vi "Main.vi"(11 "Module Admin":refnum<class "Delacor_lib_QMH_Module Admin.lvclass">) -> ()   [LabVIEW 2021, in "TDMS.lvlib"]
doc: "This template is based off of the Queued Message Handler design pattern and the Queued Message Handler project template that ships with LabVIEW.\n\nThe main difference is that the queue is private to this module and communication between modules is performed via Broadcast and Request events.\n\nRequest events are wrapped in public API methods and are handled in the Event Handling Loop (EHL) of this VI. Any module can register for Broadcast events sent by this module. The EHL generates messages based on user interface actions.\n\nThe Message Handling Loop (MHL) processes messages generated by the EHL, or by other messages. The messages are string values, so new messages can be added easily to the Message Cases case structure in the MHL. Each message cluster can also provide an optional value for Message Data, which is a variant that can be converted to whatever message-specific data is required.\n_____\nBased on DQMH Project Template 7.0.1.1316."
uses:
  TDMS.lvlib
  <vilib>/Delacor/Delacor QMH/Libraries/Module Admin_class/Delacor_lib_QMH_Module Admin.lvclass
  Module Data--cluster.ctl
  Stop Argument--cluster.ctl
  <vilib>/Delacor/Delacor QMH/Libraries/Message Queue_class/Delacor_lib_QMH_Message Queue.lvclass/Delacor_lib_QMH_Message Queue.ctl
  <vilib>/Delacor/Delacor QMH/Libraries/Module Admin_class/Delacor_lib_QMH_Module Admin.lvclass/Delacor_lib_QMH_Module Admin.ctl
  Write Data Argument--cluster.ctl
  RT Main/Data Cluster.ctl
  <vilib>/Delacor/Delacor QMH/Libraries/Message Queue_class/Delacor_lib_QMH_Enqueue Message (Single).vi
  <vilib>/Delacor/Delacor QMH/Libraries/Module Admin_class/Delacor_lib_QMH_Get External Launch.vi
  <vilib>/Delacor/Delacor QMH/Libraries/Message Queue_class/Delacor_lib_QMH_Message Queue.lvclass
  RT Main/RT Main.lvlib
  <vilib>/WebDAVClient/NI_WebDAV.lvlib
  <vilib>/WebDAVClient/Advanced/Get File.vi
panel:
  out "error out":errorcluster
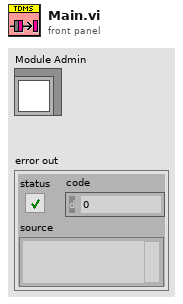
[diagram p1: front panel]
types:
  T1 = typedef "TDMS.lvlib/Request Events--cluster.ctl" = cluster{"Stop Module":refnum<user-event>, "Show Panel":refnum<user-event>, "Hide Panel":refnum<user-event>, "Get Module Execution Status":refnum<user-event>, "Show Diagram":refnum<user-event>, "Create TDMS File":refnum<user-event>, "Close TDMS File":refnum<user-event>, "Write Data":refnum<user-event>, "Private.Write Data to File":refnum<user-event>}
  T2 = typedef "TDMS.lvlib/Module Data--cluster.ctl" = cluster{"Status":string, "Path":path, "tdms file Ref":refnum<k34>}
  T3 = enum32{"invalid lock state", "Not Locked", "Locked (No Password)", "Password-protected"}
  T4 = typedef "TDMS.lvlib/Stop Argument--cluster.ctl" = cluster{"Origin":string, "Exit via Stop Module Req?":bool, "Wait for Module to stop?":bool}
  T5 = typedef "TDMS.lvlib/Write Data Argument--cluster.ctl" = cluster{"Data":T6[]}
  T6 = typedef "RT Main.lvlib/Data Cluster.ctl" = cluster{"Analog Input":dbl[], "Digital Inputs":bool[], "U32":u32[]}
  T7 = enum16{"open", "open or create", "create or replace", "create", "open (read-only)"}
  T8 = typedef "NI_WebDAV.lvlib/SessionHandle.ctl" = refnum<k1>
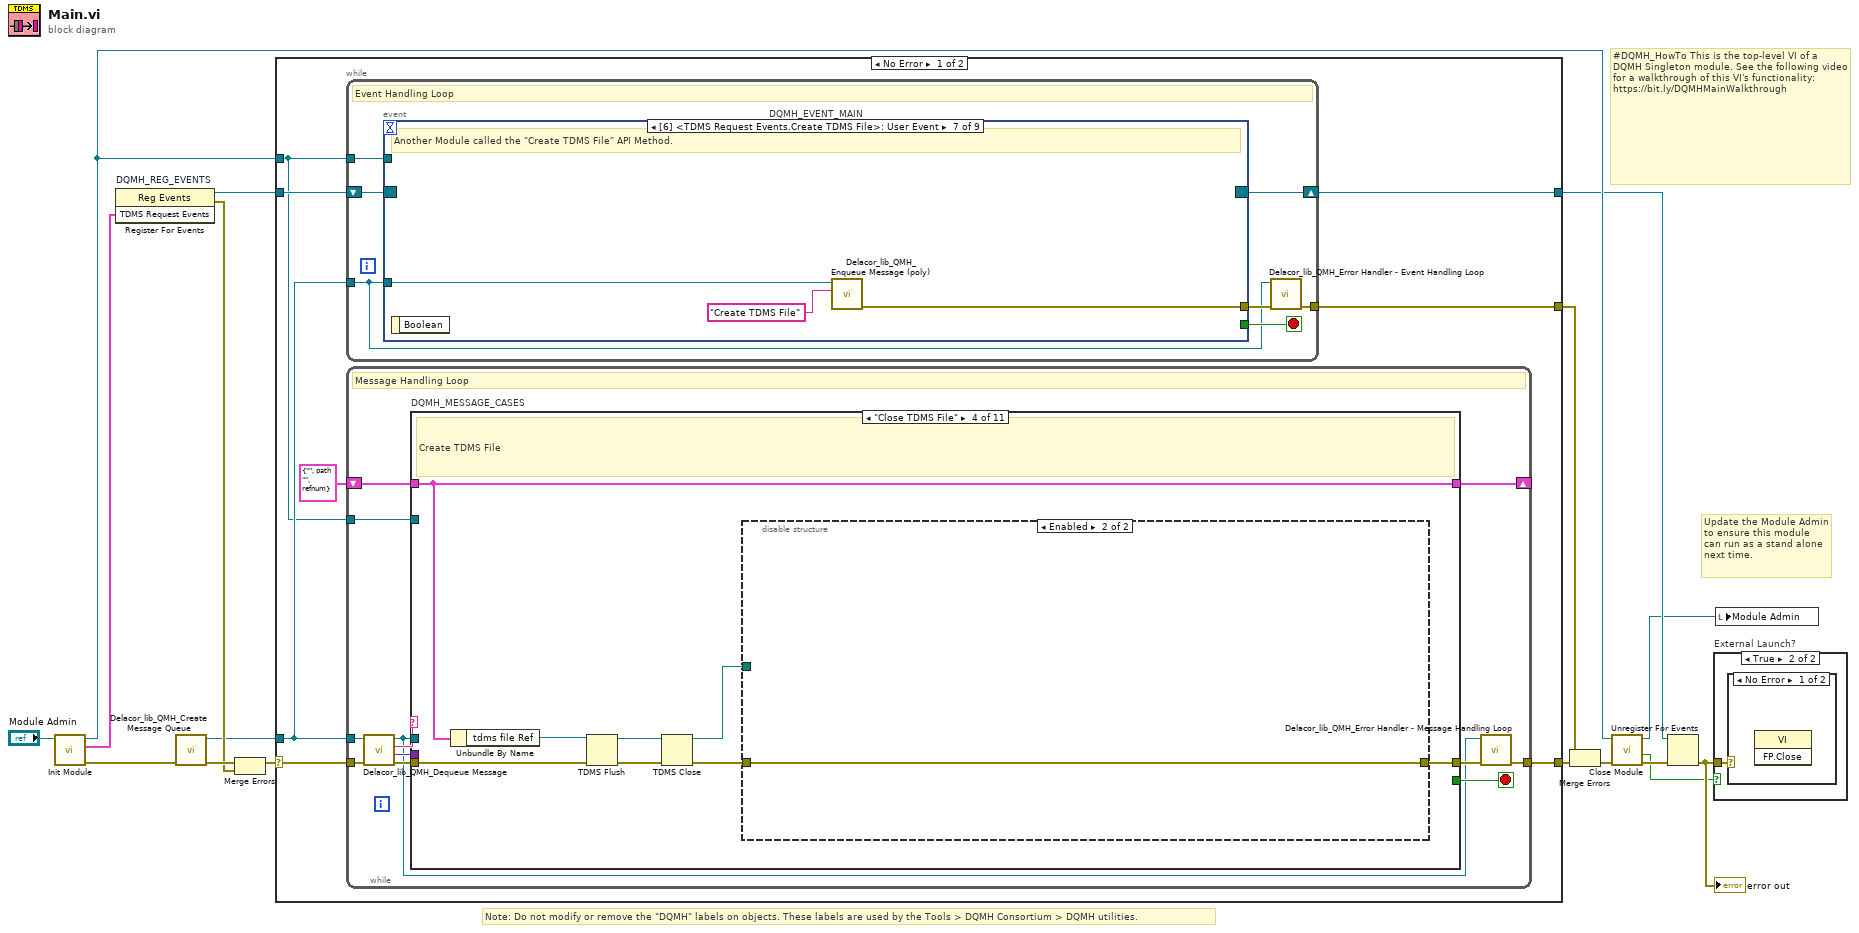
[diagram p0: block diagram]
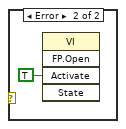
[diagram p3: hidden frame]
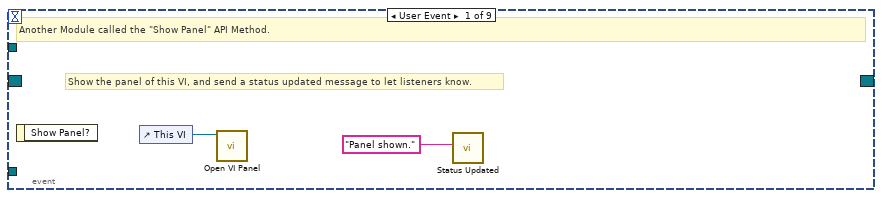
[diagram p4: hidden frame]
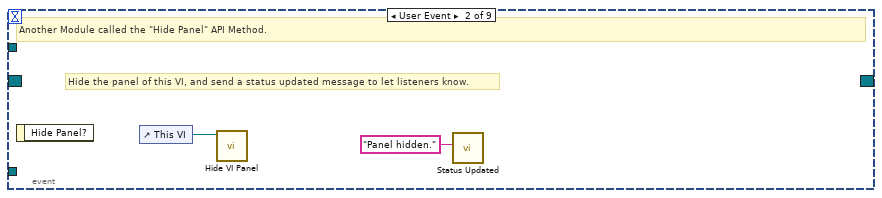
[diagram p5: hidden frame]
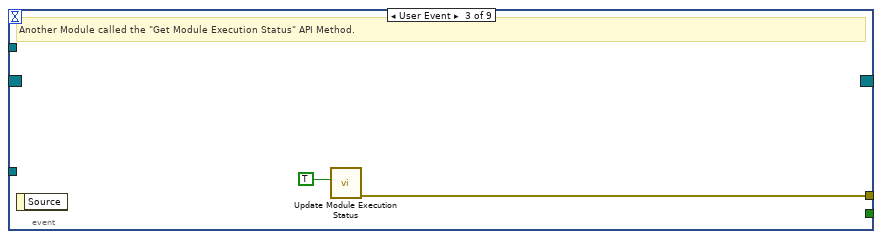
[diagram p6: hidden frame]
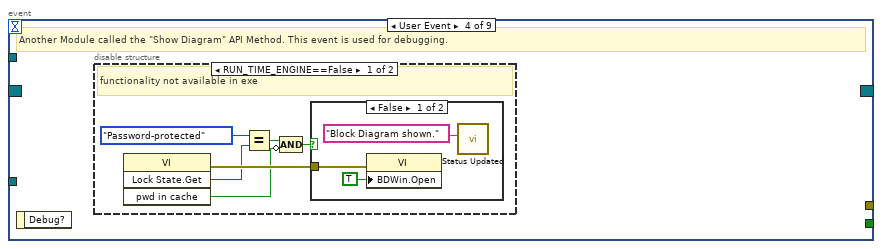
[diagram p7: hidden frame]
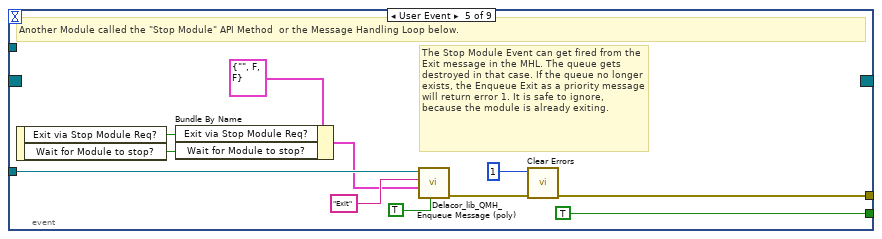
[diagram p10: hidden frame]
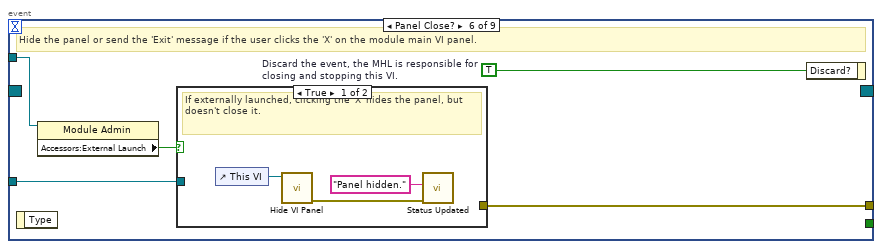
[diagram p11: hidden frame]
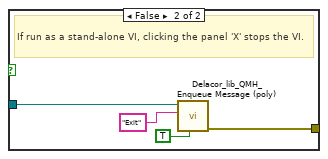
[diagram p12: hidden frame]
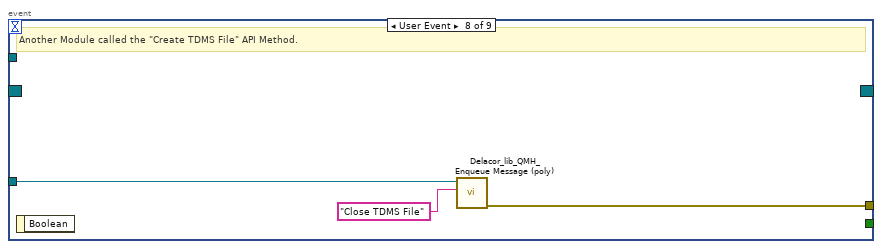
[diagram p13: hidden frame]
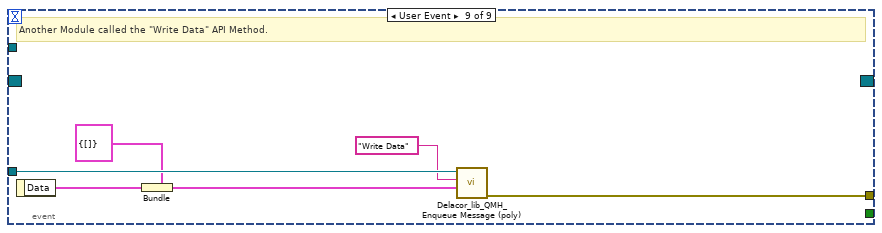
[diagram p14: hidden frame]
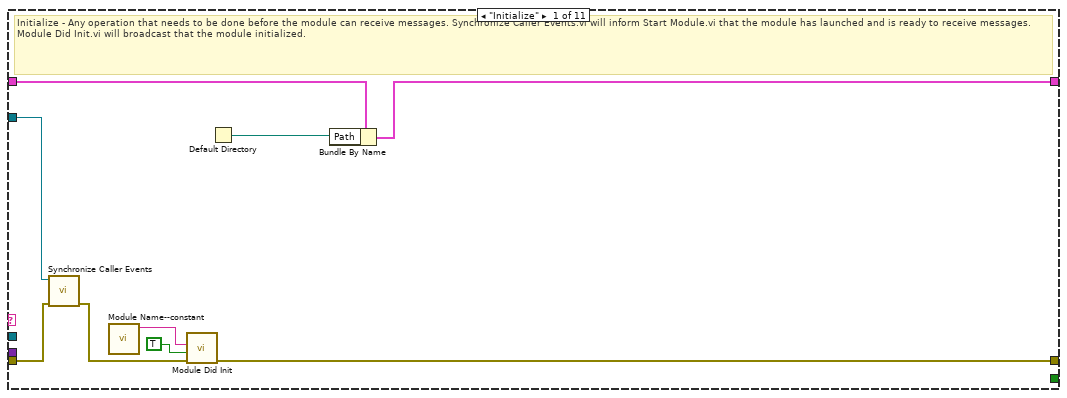
[diagram p15: hidden frame]
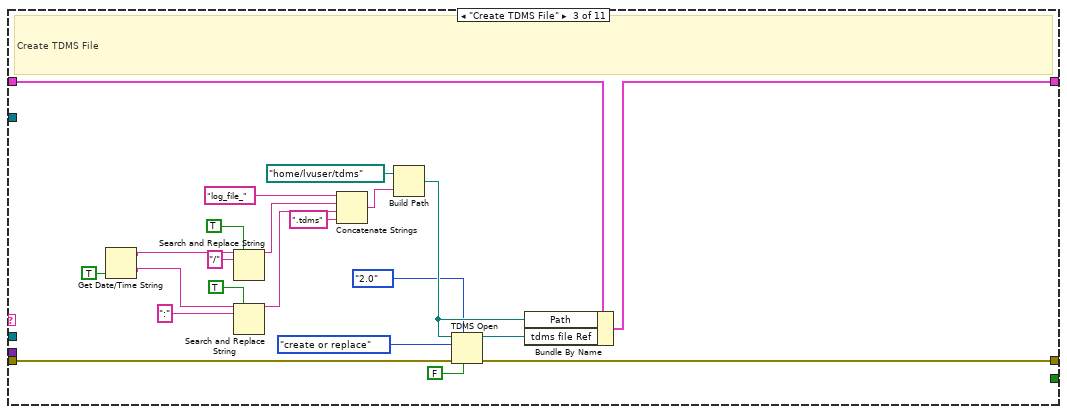
[diagram p17: hidden frame]
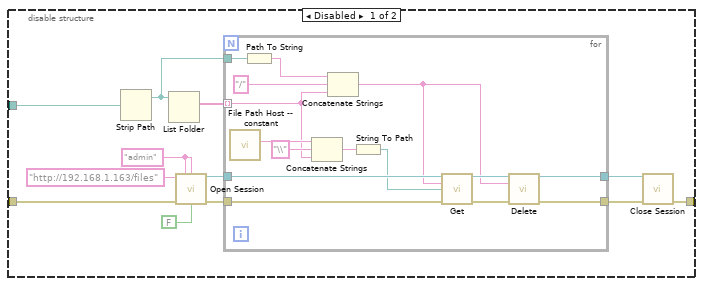
[diagram p18: hidden frame]
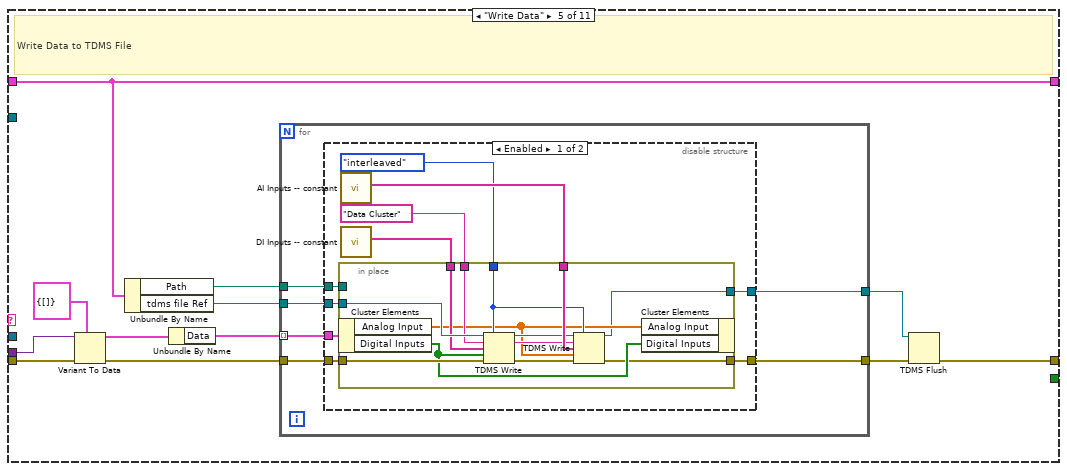
[diagram p19: hidden frame]
diagram:
  # "#DQMH_HowTo This is the top-level VI of a DQMH Singleton module. See the following video for a walkthrough of this VI's functionality: https://bit.ly/DQMHMainWalkthrough"
  # "Note: Do not modify or remove the \"DQMH\" labels on objects. These labels are used by the Tools > DQMH Consortium > DQMH utilities."
  # "Update the Module Admin to ensure this module can run as a stand alone next time."
  n1 = call "Init Module.vi"("Singleton Module Admin in"="Module Admin") -> ("error out"=w16:errorcluster, "TDMS Request Events"=w1:T1, "Singleton Module Admin out"=w8:refnum<class "Delacor_lib_QMH_Module Admin.lvclass">)  [unwired: 8 in]
  n2 = register-events "DQMH_REG_EVENTS"(w1) -> (reference out=w6:refnum<event-registration>, error out=w9:errorcluster)  [unwired: 2 in]
  n3 = call <vilib>:"Delacor_lib_QMH_Create Message Queue.vi"("error in"=w16) -> ("error out"=w11:errorcluster, "Message Queue"=w5:refnum<class "Delacor_lib_QMH_Message Queue.lvclass">)  [unwired: 9 in]
  n4 = Merge Errors(w11, w9) -> (w10:errorcluster)
  n5 = case shown="No Error" w10 {
    selector: w10 -> [w23 w269]
    tunnel: [w25 w268] -> w17
    tunnel: [w22 w267] -> w7
    tunnel: w6 -> [w20 w267]
    tunnel: w5 -> [w19 w262]
    tunnel: [w24 _] -> w14
    tunnel: w8 -> [w18 w263]
    frame No Error {
      n6 = while {
        tunnel: w19 -> [w26]
        shift-right: [w29] -> w22
        shift-left: w20 -> [w30]
        tunnel: [w31] -> w24
        tunnel: w18 -> [w27]
        stop <- w28 stop-if-true
        # "Event Handling Loop"
        n7 = event "DQMH_EVENT_MAIN" shown="[6] <TDMS Request Events.Create TDMS File>: User Event" {
          selector: w30 -> [_ _ _ _ _ _ _ _ _]
          dyn-events: [_ _ _ _ _ _ _ _ _] -> w29
          timeout: _ -> [_ _ _ _ _ _ _ _ _]
          tunnel: [_ _ _ _ TRUE ("Discard?") _ _ _ _] -> w28
          tunnel: w26 -> [_ _ _ _ w54 w61 w73 w76 w82]
          tunnel: [_ _ w38 _ w57 w63 w71 w74 w77] -> w32
          tunnel: w27 -> [_ _ _ _ _ w60 _ _ _]
          event User Event {
            # "Show the panel of this VI, and send a status updated message to let listeners know."
            # "Another Module called the \"Show Panel\" API Method."
            n8 = event-data() -> ()  [unwired: 1 in, 1 out]
            n9 = control-ref of="This VI"() -> (w34:refnum<vi>)
            n10 = call "Open VI Panel.vi"("VI"=w34) -> ()  [unwired: 10 in, 1 out]
            n11 = call "Status Updated.vi"("Status"="Panel shown." ("format string")) -> ()  [unwired: 10 in, 1 out]
          }
          event User Event {
            # "Hide the panel of this VI, and send a status updated message to let listeners know."
            # "Another Module called the \"Hide Panel\" API Method."
            n12 = event-data() -> ()  [unwired: 1 in, 1 out]
            n13 = control-ref of="This VI"() -> (w36:refnum<vi>)
            n14 = call "Hide VI Panel.vi"("VI"=w36) -> ()  [unwired: 10 in, 1 out]
            n15 = call "Status Updated.vi"("Status"="Panel hidden." ("format string")) -> ()  [unwired: 10 in, 1 out]
          }
          event User Event {
            # "Another Module called the \"Get Module Execution Status\" API Method."
            n16 = event-data() -> ()  [unwired: 1 in, 1 out]
            n17 = call "Update Module Execution Status.vi"("Running?"=TRUE) -> ("error out"=w38:errorcluster)  [unwired: 10 in]
          }
          event User Event {
            # "Another Module called the \"Show Diagram\" API Method. This event is used for debugging."
            n18 = event-data() -> ()  [unwired: 1 in, 1 out]
            n19 = disable-structure shown="RUN_TIME_ENGINE==False" {
              frame condition #0 (active) {
                # "functionality not available in exe"
                n20 = invoke on="Invoke Node" class="VI" method="Lock State.Get"() -> (error out=w44:errorcluster, "Get Lock State"=w43:T3, "pwd in cache"=w40:bool)  [unwired: 4 in, 1 out]
                n21 = Equal?(x=T3."Password-protected", y=w43) -> (x = y?=w41:bool)
                n22 = Compound Arithmetic op=AND(w41, invert w40) -> (w39:bool)
                n23 = case shown="False" w39 {
                  tunnel: w44 -> [w47 _]
                  frame False {
                    n24 = property on="Property Node" class="VI"(error in=w47, "BDWin.Open"=TRUE ("Block Diagram Window:Open")) -> ()  [unwired: 1 in, 2 out]
                    n25 = call "Status Updated.vi"("Status"="Block Diagram shown." ("format string")) -> ()  [unwired: 10 in, 1 out]
                  }
                  frame True {
                    # "Password-protected VI, and the password is not in the cache. Do not show the diagram."
                  }
                }
              }
              frame condition #1 {
              }
            }
          }
          event User Event {
            # "The Stop Module Event can get fired from the Exit message in the MHL. The queue gets destroyed in that case. If the queue no longer exists, the Enqueue Exit as a priority message will return error 1. It is safe to ignore, because the module is already exiting."
            # "Another Module called the \"Stop Module\" API Method  or the Message Handling Loop below."
            n26 = event-data() -> ("Exit via Stop Module Req?"=w50:bool, "Wait for Module to stop?"=w49:bool)  [unwired: 1 in]
            n27 = Bundle By Name(cluster=T4 {"Origin"="", "Exit via Stop Module Req?"=FALSE, "Wait for Module to stop?"=FALSE} ("Stop Argument"), "Exit via Stop Module Req?"=w50, "Wait for Module to stop?"=w49) -> (w48:T4)
            n28 = call-poly <vilib>:"Delacor_lib_QMH_Enqueue Message (poly).vi"("Priority Message? (F)"=TRUE, "Message Data"=w48, "Message"="Exit", "Message Queue in"=w54) -> ("error out"=w58:errorcluster)  [unwired: 6 in, 1 out]
            n29 = call <vilib>:"Clear Errors.vi"("error in (no error)"=w58, "specific error code to clear (0: all)"=1) -> ("error out"=w57:errorcluster)  [unwired: 4 in, 1 out]
          }
          event Panel Close? {
            w62 = TRUE  # Discard the event, the MHL is responsible for closing and stopping this VI.
            # "Hide the panel or send the 'Exit' message if the user clicks the 'X' on the module main VI panel."
            n30 = event-data() -> ()  [unwired: 1 in, 1 out]
            n31 = property on="Property Node" class="Module Admin"(reference=w60) -> ("Accessors:External Launch"=w59:bool)  [unwired: 1 in, 2 out]
            n32 = case shown="True" w59 {
              tunnel: w61 -> [_ w69]
              tunnel: [_ w70] -> w63
              frame True {
                # "If externally launched, clicking the 'X' hides the panel, but doesn't close it."
                n33 = control-ref of="This VI"() -> (w66:refnum<vi>)
                n34 = call "Hide VI Panel.vi"("VI"=w66) -> ("error out"=w64:errorcluster)  [unwired: 10 in]
                n35 = call "Status Updated.vi"("error in"=w64, "Status"="Panel hidden." ("format string")) -> ()  [unwired: 9 in, 1 out]
              }
              frame False {
                # "If run as a stand-alone VI, clicking the panel 'X' stops the VI."
                n36 = call-poly <vilib>:"Delacor_lib_QMH_Enqueue Message (poly).vi"("Priority Message? (F)"=TRUE, "Message"="Exit", "Message Queue in"=w69) -> ("error out"=w70:errorcluster)  [unwired: 7 in, 1 out]
              }
            }
            n37 = event-data ("Event Filter Node")("Discard?"=w62) -> ()  [unwired: 1 in, 1 out]
          }
          event User Event {
            # "Another Module called the \"Create TDMS File\" API Method."
            n38 = event-data() -> ()  [unwired: 1 in, 1 out]
            n39 = call-poly <vilib>:"Delacor_lib_QMH_Enqueue Message (poly).vi"("Message"="Create TDMS File", "Message Queue in"=w73) -> ("error out"=w71:errorcluster)  [unwired: 8 in, 1 out]
          }
          event User Event {
            # "Another Module called the \"Create TDMS File\" API Method."
            n40 = event-data() -> ()  [unwired: 1 in, 1 out]
            n41 = call-poly <vilib>:"Delacor_lib_QMH_Enqueue Message (poly).vi"("Message"="Close TDMS File", "Message Queue in"=w76) -> ("error out"=w74:errorcluster)  [unwired: 8 in, 1 out]
          }
          event User Event {
            # "Another Module called the \"Write Data\" API Method."
            n42 = event-data() -> ("Data"=w78:T6[])  [unwired: 1 in]
            n43 = Bundle(cluster=T5 {"Data"=[]} ("Write Data Argument"), "Data"=w78) -> (w79:T5)
            n44 = call-poly <vilib>:"Delacor_lib_QMH_Enqueue Message (poly).vi"("Message Data"=w79, "Message"="Write Data", "Message Queue in"=w82) -> ("error out"=w77:errorcluster)  [unwired: 7 in, 1 out]
          }
        }
        n45 = call-dynamic "Delacor_lib_QMH_Error Handler - Event Handling Loop.vi"("error in"=w32, "Message Queue in"=w26) -> ("dup error in"=w31:errorcluster)  [unwired: 8 in, 1 out]
      }
      n46 = while {
        tunnel: w19 -> [w83]
        shift-right: [w91] -> _
        shift-left: T2 {"Status"="", "Path"=path "", "tdms file Ref"=refnum} ("Data Cluster") -> [w92]
        tunnel: w23 -> [w94]
        tunnel: [w86] -> w25
        tunnel: w18 -> [w87]
        stop <- w90 stop-if-true
        # "Message Handling Loop"
        n47 = call-dynamic "Delacor_lib_QMH_Dequeue Message.vi"("error in"=w94, "Message Queue in"=w83) -> ("error out"=w93:errorcluster, "Message Data"=w88:variant, "Message"=w89:string, "Message Queue out"=w84:refnum<class "Delacor_lib_QMH_Message Queue.lvclass">)  [unwired: 6 in]
        n48 = case "DQMH_MESSAGE_CASES" shown="\"Close TDMS File\"" w89 {
          selector: w89 -> [_ _ _ _ _ _ _ _ _ _ w257]
          tunnel: w84 -> [_ _ _ _ _ _ _ _ w223 w245 _]
          tunnel: w93 -> [w103 w105 w126 w129 w175 w208 w210 w219 w230 w251 w260]
          tunnel: [w98 w105 w127 w132 w166 w207 w210 w218 w226 w246 w261] -> w85
          tunnel: w92 -> [w96 w104 w111 w135 w170 w206 w209 w216 w225 w244 w258]
          tunnel: [w97 w104 w112 w135 w170 w206 w209 w216 w225 w244 w258] -> w91
          tunnel: [_ _ _ _ _ _ _ _ _ w243 _] -> w90
          tunnel: w88 -> [_ _ _ _ w174 _ _ _ w224 w242 _]
          tunnel: w87 -> [w101 _ _ _ _ _ _ _ w222 w237 _]
          frame "Initialize" {
            # "Initialize - Any operation that needs to be done before the module can receive messages. Synchronize Caller Events.vi will inform Start Module.vi that the module has launched and is ready to receive messages. Module Did Init.vi will broadcast that the module initialized."
            n49 = call "Synchronize Caller Events.vi"("error in"=w103, "Singleton Module Admin in"=w101) -> ("error out"=w102:errorcluster)  [unwired: 8 in, 1 out]
            n50 = call "Module Name--constant.vi"() -> ("Module Name"=w99:string)  [unwired: 11 in]
            n51 = call "Module Did Init.vi"("error in"=w102, "Initialized?"=TRUE, "Origin"=w99) -> ("error out"=w98:errorcluster)  [unwired: 8 in]
            n52 = Default Directory() -> (w95:path)
            n53 = Bundle By Name(cluster=w96, "Path"=w95) -> (w97:T2)
          }
          frame "---Module Specific---" {
            # "Separator -- The following cases handle messages specific to this Module."
          }
          frame "Create TDMS File" {
            # "Create TDMS File"
            n54 = Get Date/Time String(want seconds? (F)=TRUE) -> (date string=w118:string, time string=w117:string)  [unwired: 2 in]
            n55 = Search and Replace String(replace all?=TRUE ("replace all? (F)"), input string=w118, search string="/") -> (result string=w116:string)  [unwired: 5 in, 3 out]
            n56 = Search and Replace String(replace all?=TRUE ("replace all? (F)"), input string=w117, search string=":") -> (result string=w115:string)  [unwired: 5 in, 3 out]
            n57 = Concatenate Strings("log_file_", w116, w115, ".tdms" ("string")) -> (w113:string)
            n58 = Build Path(base path=path "/home/lvuser/tdms", name or relative path=w113) -> (appended path=w108:path)
            n59 = TDMS Open(6:FALSE ("disable buffering? (T)"), 7:enum16{"1.0", "2.0"}."2.0" ("file format version (2.0)"), 8:w126, 10:T7."create or replace" ("operation (0:open)"), 11:w108) -> (0:w127:errorcluster, 3:w125:refnum<k34>)  [unwired: 2 in]
            n60 = Bundle By Name(cluster=w111, "Path"=w108, "tdms file Ref"=w125) -> (w112:T2)
          }
          frame "Close TDMS File" {
            # "Create TDMS File"
            n61 = Unbundle By Name(w135) -> ("tdms file Ref"=w131:refnum<k34>)
            n62 = TDMS Flush(4:w129, 7:w131) -> (0:w128:errorcluster, 3:w130:refnum<k34>)
            n63 = TDMS Close(8:w128, 11:w130) -> (0:w133:errorcluster, 3:w134:path)
            n64 = disable-structure shown="Enabled" {
              disable-tunnel: w134 -> [w147 _]
              disable-tunnel: w133 -> [w145 w163]
              disable-tunnel: [w136 w163] -> w132
              frame Disabled {
                w142 = "admin" ("username")
                n65 = Strip Path(path=w147) -> (stripped path=w139:path)  [unwired: 1 out]
                n66 = List Folder(path=w139) -> (filenames=w146:string[])  [unwired: 3 in, 3 out]
                n67 = call <vilib>:"Open Session.vi"("host uri prefix"="http://192.168.1.163/files", "username"=w142, "password"=w142, "error in (no error)"=w145, "verify server?"=FALSE) -> ("session handle out"=w143:T8, "error out"=w144:errorcluster)  [unwired: 9 in]
                n68 = for {
                  tunnel: w146 -> [w150] mode=indexing
                  tunnel: w144 -> [w158]
                  tunnel: w143 -> [w162]
                  tunnel: w139 -> [w161]
                  tunnel: [w154] -> w138
                  tunnel: [w153] -> w137
                  n69 = call "File Path Host -- constant.vi"() -> ("File Path Control"=w152:string)  [unwired: 11 in]
                  n70 = Path To String(path=w161) -> (string=w160:string)
                  n71 = Concatenate Strings(w152, "\\" ("string"), w150) -> (w149:string)
                  n72 = Concatenate Strings(w160, "/" ("string"), w150) -> (w156:string)
                  n73 = String To Path(string=w149) -> (path=w148:path)
                  n74 = call-poly <vilib>:"Get.vi"("session handle"=w162, "relative uri"=w156, "local file path"=w148, "error in (no error)"=w158) -> ("session handle out"=w157:T8, "error out"=w155:errorcluster)  [unwired: 9 in, 1 out]
                  n75 = call <vilib>:"Delete.vi"("session handle"=w157, "relative uri"=w156, "error in (no error)"=w155) -> ("session handle out"=w154:T8, "error out"=w153:errorcluster)  [unwired: 11 in]
                }
                n76 = call <vilib>:"Close Session.vi"("session handle"=w138, "error in (no error)"=w137) -> ("error out"=w136:errorcluster)  [unwired: 13 in]
              }
              frame Enabled {
              }
            }
          }
          frame "Write Data" {
            # "Write Data to TDMS File"
            n77 = Variant To Data(error in=w175, type=T5 {"Data"=[]} ("Write Data Argument"), Variant=w174) -> (data=w172:T5, error out=w171:errorcluster)
            n78 = Unbundle By Name(w170) -> ("Path"=w167:path, "tdms file Ref"=w168:refnum<k34>)
            n79 = Unbundle By Name(w172) -> ("Data"=w169:T6[])
            n80 = for {
              tunnel: w171 -> [w181]
              tunnel: w169 -> [w178] mode=indexing
              tunnel: w168 -> [w180]
              tunnel: [w179] -> w165
              tunnel: w167 -> [w177]
              tunnel: [w176] -> w164
              n81 = disable-structure shown="Enabled" {
                disable-tunnel: w181 -> [w191 w205]
                disable-tunnel: w180 -> [w190 _]
                disable-tunnel: [w182 w205] -> w179
                disable-tunnel: w178 -> [w185 _]
                disable-tunnel: w177 -> [w184 _]
                disable-tunnel: [w183 _] -> w176
                frame Enabled {
                  n82 = call "AI Inputs -- constant.vi"() -> ("AI Inputs"=w188:string[])  [unwired: 11 in]
                  n83 = call "DI Inputs -- constant.vi"() -> ("DI Inputs"=w189:string[])  [unwired: 11 in]
                  n84 = in-place {
                    in-place-border: w191 -> [w204]
                    in-place-border: w190 -> [w203]
                    in-place-border: w189 -> [w201]
                    in-place-border: w188 -> [w200]
                    in-place-border: enum16{"decimated", "interleaved"}."interleaved" ("data layout (0:decimated)") -> [w198]
                    in-place-border: "Data Cluster" ("group name in (Untitled)") -> [w197]
                    in-place-border: w184 -> [_]
                    in-place-border: [w193] -> w183
                    in-place-border: [w192] -> w182
                    n85 = in-place-cluster #1(w185) -> ("Analog Input"=w195:dbl[], "Digital Inputs"=w194:bool[])
                    n86 = TDMS Write(0:w203, 1:w198, 5:w197, 7:w201, 9:w194, 11:w204) -> (4:w199:refnum<k34>, 6:w196:string, 15:w202:errorcluster)  [unwired: 1 out]
                    n87 = TDMS Write(0:w199, 1:w198, 5:w196, 7:w200, 9:w195, 11:w202) -> (4:w193:refnum<k34>, 15:w192:errorcluster)  [unwired: 2 out]
                    n88 = in-place-cluster #1("Analog Input"=w195, "Digital Inputs"=w194) -> ()  [unwired: 1 out]
                  }
                }
                frame Disabled {
                }
              }
            }
            n89 = TDMS Flush(4:w165, 7:w164) -> (0:w166:errorcluster)  [unwired: 1 out]
          }
          frame "---Copy This Frame---" {
            # "Duplicate this frame when creating new messages.  Change this comment in the duplicated frame to describe this message."
            n90 = Merge Errors(w208) -> (w207:errorcluster)
          }
          frame "---Exit and Error Handling---" {
            # "Separator - The following cases handle errors and exit messages."
          }
          frame "Simulate MHL Error" {
            # "#DQMH_HowTo The 'Simulate MHL Error' button  illustrates how the MHL handles errors. This event is instructional in nature and can be removed."
            # "Simulate an error occurring at the MHL"
            n91 = call "Module Name--constant.vi"() -> ("Module Name"=w212:string)  [unwired: 11 in]
            n92 = Format Into String(format string="Simulated error originating at Message Handling Loop in %s", w212) -> (resulting string=w213:string)  [unwired: 2 in, 1 out]
            n93 = call <vilib>:"Error Cluster From Error Code.vi"("show call chain? (False)"=TRUE, "error message (\"\")"=w213, "error code (0)"=5001) -> ("error out"=w217:errorcluster)  [unwired: 6 in]
            n94 = Merge Errors(w219, w217) -> (w218:errorcluster)
          }
          frame "Error" {
            # "#CodeRecommended - If the module is running in standalone mode (External Launch = FALSE), this code will pop up an error dialog and call the 'Exit' message if an error occurs. Add more fine-grained error management here."
            # "Error - Check the error message data and respond accordingly. This message is sent by the \"Error Handler\" VIs at the end of each loop in this application."
            n95 = property on="Property Node" class="Module Admin"(reference=w222) -> ("Accessors:External Launch"=w221:bool)  [unwired: 1 in, 2 out]
            n96 = Variant To Data(error in=w230, type=errorcluster {"status"=FALSE, "code"=0, "source"=""} ("error constant"), Variant=w224) -> (data=w220:errorcluster, error out=w228:errorcluster)
            n97 = local write "error out"(w220) -> ()
            n98 = call "Error Reported.vi"("Error"=w220) -> ()  [unwired: 10 in, 1 out]
            n99 = case shown="False" w221 {
              tunnel: [w235 _] -> w227
              tunnel: w223 -> [w233 _]
              tunnel: w220 -> [w234 _]
              frame False {
                n100 = disable-structure shown="Default" {
                  disable-tunnel: w234 -> [w236 _]
                  frame condition #0 (active) {
                    # "If the module is running standalone, then pop up an error dialog and call the \"Exit\" message."
                    n101 = call <vilib>:"Simple Error Handler.vi"("error in (no error)"=w236) -> ()  [unwired: 4 in, 5 out]
                  }
                  frame condition #1 {
                    # "To prevent the Simple Error Handler VI from being loaded (e.g. when deploying to a Real-Time target), add the Conditional Disable Symbol \"DQMH_Disable_SEH\" to your project and set it to TRUE."
                  }
                }
                n102 = call-poly <vilib>:"Delacor_lib_QMH_Enqueue Message (poly).vi"("Priority Message? (F)"=TRUE, "Message"="Exit", "Message Queue in"=w233) -> ("error out"=w235:errorcluster)  [unwired: 7 in, 1 out]
              }
              frame True {
                # "If the module was launched externally, calling the Error Reported broadcast VI is the only action performed by the \"Error\" message. The module's caller can then process the error appropriately."
              }
            }
            n103 = Merge Errors(w228, w227) -> (w226:errorcluster)
          }
          frame "Exit" {
            w241 = 91  # 91: not all Exit messages will have an argument
            w243 = TRUE  # Stop the VI
            # "Release the message queue reference"
            # "Exit - Exit the application."
            n104 = Variant To Data(error in=w251, type=T4 {"Origin"="", "Exit via Stop Module Req?"=FALSE, "Wait for Module to stop?"=FALSE} ("Stop Argument"), Variant=w242) -> (data=w239:T4, error out=w248:errorcluster)
            n105 = call <vilib>:"Clear Errors.vi"("error in (no error)"=w248, "specific error code to clear (0: all)"=w241) -> ("error out"=w250:errorcluster)  [unwired: 4 in, 1 out]
            n106 = control-ref of="This VI"() -> (w238:refnum<vi>)
            n107 = call-dynamic "Delacor_lib_QMH_Release Message Queue.vi"("error in"=w250, "Message Queue"=w245) -> ("error out"=w249:errorcluster)  [unwired: 9 in]
            n108 = call "Handle Exit.vi"("Stop Argument"=w239, "Admin in"=w237, "VI reference"=w238) -> ("error out"=w247:errorcluster)  [unwired: 7 in, 1 out]
            n109 = Merge Errors(w249, w247) -> (w246:errorcluster)
            n110 = call "Error Reported.vi"("Error"=w246) -> ()  [unwired: 10 in, 1 out]
          }
          frame Default {
            # "'Default' case only runs if there is a message that isn't defined in any of the other cases.  Output a programming error."
            n111 = call "Module Name--constant.vi"() -> ("Module Name"=w256:string)  [unwired: 11 in]
            n112 = Format Into String(format string="The invalid message string \"%s\" was received in the Message Handling Loop for module \"%s\".", w257, w256) -> (resulting string=w252:string)  [unwired: 2 in, 1 out]
            n113 = call <vilib>:"Error Cluster From Error Code.vi"("show call chain? (False)"=TRUE, "error message (\"\")"=w252, "error code (0)"=1) -> ("error out"=w259:errorcluster)  [unwired: 6 in]
            n114 = Merge Errors(w260, w259) -> (w261:errorcluster)
          }
        }
        n115 = call-dynamic "Delacor_lib_QMH_Error Handler - Message Handling Loop.vi"("error in"=w85, "Message Queue in"=w84) -> ("dup error in"=w86:errorcluster)  [unwired: 8 in, 1 out]
      }
    }
    frame Error {
      # "Synchronize Caller Events.vi will inform Start Module.vi that the module has launched and will let the code calling Start Module.vi register for broadcasts and would permit the caller receive the broadcast that an error occurred at launch time."
      n116 = call-dynamic "Delacor_lib_QMH_Release Message Queue.vi"("error in"=w269, "Message Queue"=w262) -> ("error out"=w268:errorcluster)  [unwired: 9 in]
      n117 = call "Synchronize Caller Events.vi"("Singleton Module Admin in"=w263) -> ("error out"=w270:errorcluster)  [unwired: 9 in, 1 out]
      n118 = call "Module Name--constant.vi"() -> ("Module Name"=w266:string)  [unwired: 11 in]
      n119 = Format Into String(format string="An error occurred during initialization. %s is no longer running.", w266) -> (resulting string=w264:string)  [unwired: 2 in, 1 out]
      n120 = Merge Errors(w268, w270) -> (w271:errorcluster)
      n121 = call "Error Reported.vi"("Additional Information"=w264, "Error"=w271) -> ()  [unwired: 9 in, 1 out]
    }
  }
  n122 = Merge Errors(w14, w17) -> (w13:errorcluster)
  n123 = call "Close Module.vi"("error in"=w13, "Module Admin in"=w8) -> ("error out"=w15:errorcluster, "External Launch"=w2:bool, "Module Admin out"=w3:refnum<class "Delacor_lib_QMH_Module Admin.lvclass">)  [unwired: 7 in]
  n124 = Unregister For Events(event registration refnum=w7, error in=w15) -> (error out=w12:errorcluster)
  "error out" <- w12
  n125 = case "External Launch?" shown="True" w2 {
    tunnel: w12 -> [_ w272]
    frame False {
    }
    frame True {
      n126 = case shown="No Error" w272 {
        frame No Error {
          n127 = invoke on="Invoke Node" class="VI" method="FP.Close"() -> ()  [unwired: 3 in, 3 out]
        }
        frame Error {
          n128 = invoke on="Invoke Node" class="VI" method="FP.Open"("Activate"=TRUE ("Activate?")) -> ()  [unwired: 4 in, 5 out]
        }
      }
    }
  }
  n129 = local write "Module Admin"(w3) -> ()
